vi "Refresh All Nodes.vi"(8 "error in (no error)":errorcluster, 10 "All Node Tags":string[](array[string])) -> (0 "error out":errorcluster)   [LabVIEW 2013, in "Standard Editor.lvlib"]
uses:
  Standard Editor.lvlib
  Configuration Editor/Classes/Module editor node/module editor node.lvclass
  Configuration Editor/Classes/Engine Parent/read engine configuration.vi
  Configuration Editor/Classes/Engine Parent/write engine configuration.vi
  <vilib>/NI/Module Execution Interface/Engine Configuration/engine configuration.lvclass
  <vilib>/NI/Configuration Framework/Node/NISE_CEF_Node.lvclass
  Configuration Editor/Classes/Engine Parent/Engine Parent Editor Node.lvclass
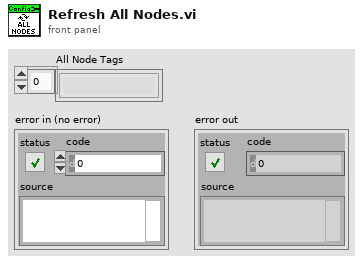
[diagram p1: front panel]
types:
  T1 = typedef "NISE_CEF_Node.lvclass/NodeRef.ctl" = refnum<data-value>
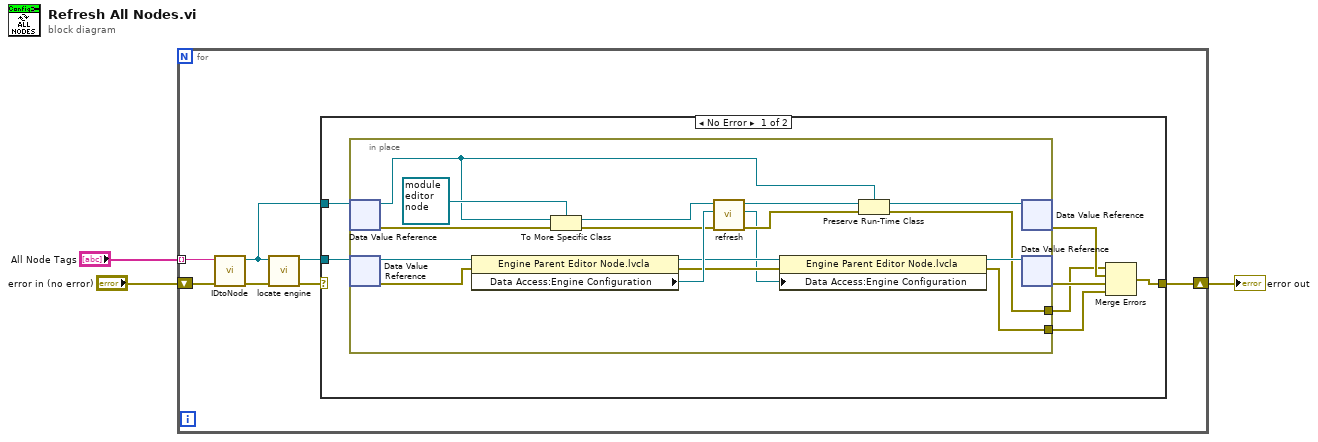
[diagram p0: block diagram]
diagram:
  n1 = for {
    tunnel: "All Node Tags" -> [w10] mode=indexing
    shift-right: [w4] -> w1
    shift-left: "error in (no error)" -> [w9]
    n2 = call <vilib>:"IDtoNode.vi"("error in"=w9, "ID"=w10) -> ("error out"=w8:errorcluster, "node ref"=w6:T1)  [unwired: 7 in, 1 out]
    n3 = call "locate engine.vi"("error in"=w8, "component"=w6) -> ("error out"=w5:errorcluster, "engine"=w7:refnum<data-value>)  [unwired: 8 in]
    n4 = case shown="No Error" w5 {
      selector: w5 -> [_ w35]
      tunnel: w7 -> [w17 _]
      tunnel: w6 -> [w16 _]
      tunnel: [w11 w35] -> w4
      frame No Error {
        n5 = in-place {
          in-place-border: [w25] -> w15
          in-place-border: [w20] -> w12
          n6 = in-place-dvr #1(w16) -> (w23:refnum<class "NISE_CEF_Node.lvclass">, w34:errorcluster)
          n7 = in-place-dvr #2(w17) -> (w32:refnum<class "Engine Parent Editor Node.lvclass">, w27:errorcluster)
          n8 = property class="Engine Parent Editor Node.lvcla"(reference=w32, error in=w27) -> (reference out=w29:refnum<class "Engine Parent Editor Node.lvclass">, error out=w28:errorcluster, "Data Access:Engine Configuration"=w30:refnum<class "engine configuration.lvclass">)
          n9 = To More Specific Class(target class=refnum<class "module editor node.lvclass"> refnum ("Tag Editor Core:module editor node"), reference=w23, error in=w34) -> (specific class reference=w31:refnum<class "module editor node.lvclass">, error out=w19:errorcluster)
          n10 = call "refresh.vi"("error in (no error)"=w19, "Engine Configuration In"=w30, "Module Editor Node In"=w31) -> ("error out"=w21:errorcluster, "Engine Configuration Out"=w18:refnum<class "engine configuration.lvclass">, "Module Editor Node Out"=w24:refnum<class "module editor node.lvclass">)  [unwired: 6 in]
          n11 = property class="Engine Parent Editor Node.lvcla"(reference=w29, error in=w28, "Data Access:Engine Configuration"=w18) -> (reference out=w26:refnum<class "Engine Parent Editor Node.lvclass">, error out=w25:errorcluster)
          n12 = Preserve Run-Time Class(object in=w24, error in=w21, 2:w23) -> (object out=w22:refnum<class "NISE_CEF_Node.lvclass">, error out=w20:errorcluster)
          n13 = in-place-dvr #1(w22) -> (w13:errorcluster)  [unwired: 1 out]
          n14 = in-place-dvr #2(w26) -> (w14:errorcluster)  [unwired: 1 out]
        }
        n15 = Merge Errors(w12, w13, w14, w15) -> (w11:errorcluster)
      }
      frame Error {
      }
    }
  }
  "error out" <- w1
